vi "Globals.vi"() -> ()   [LabVIEW 2015, in "Impenetrable.lvclass"]
uses:
  Impenetrable.lvclass
panel:
  in  "Rain Round":i32
  in  "Current Target Gap":i32
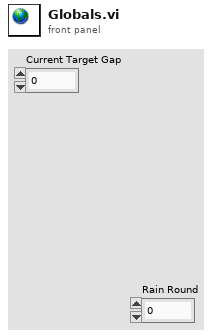
[diagram p1: front panel]
diagram:
